vi "execute.vi"(8 "error in (no error)":errorcluster, 9 "B in":refnum<class "GenericComponent.lvclass">, 10 "A in":refnum<class "GenericComponent.lvclass">, 11 "AdapterDL111013ImagingModeToScanHead in":refnum<class "AdapterDL111013ImagingModeToScanHead.lvclass">) -> (0 "error out":errorcluster, 1 "B out":refnum<class "GenericComponent.lvclass">, 2 "A out":refnum<class "GenericComponent.lvclass">, 3 "AdapterDL111013ImagingModeToScanHead out":refnum<class "AdapterDL111013ImagingModeToScanHead.lvclass">)   [LabVIEW 2010, in "AdapterDL111013ImagingModeToScanHead.lvclass"]
uses:
  AdapterDL111013ImagingModeToScanHead.lvclass
  common/classes/GenericComponent/GenericComponent/GenericComponent.lvclass
  ImagingMode/ImagingModeDL090130Frame/ImagingModeDL090130Frame/translation_mode_enum.ctl
  ScanHead/ScanHeadDL090202/ScanHeadDL090202/ScanHeadDL090202.lvclass
  ImagingMode/ImagingModeDL090130Frame/ImagingModeDL090130Frame/settings_cluster.ctl
  ImagingMode/ImagingModeDL090130Frame/ImagingModeDL090130Frame/ImagingModeDL090130Frame.lvclass
  common/xcontrols/XIntensityCompensation/XIntensityCompensation/XIntensityCompensation.xctl
  ScanHead/ScanHeadDL090202/ScanHeadDL090202/settings_cluster.ctl
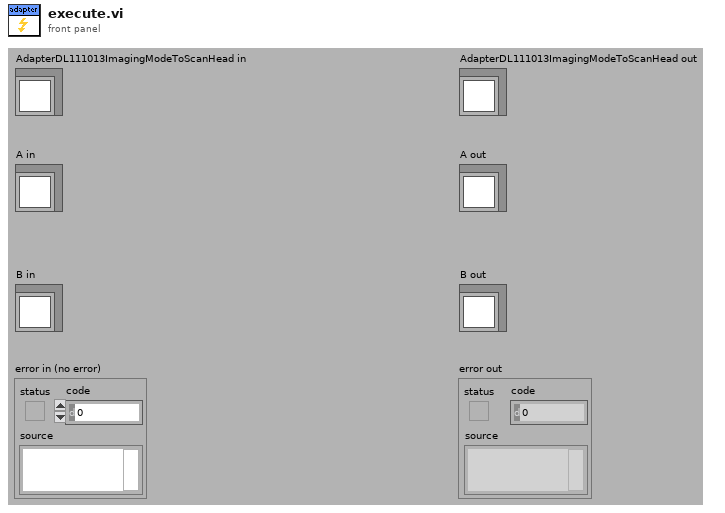
[diagram p1: front panel]
types:
  T1 = typedef "ImagingModeDL090130Frame.lvclass/translation_mode_enum.ctl" = enum16{"scanHead", "stage"}
  T2 = typedef "ImagingModeDL090130Frame.lvclass/settings_cluster.ctl" = cluster{"FrameSettings":cluster{"ResolutionX":i32, "ResolutionY":i32, "AspectRatioX":dbl, "AspectRatioY":dbl, "FrameScanRate":dbl[unit]}, "StackSettings":cluster{"Frames":i32, "AveragingRepetitions":i32, "StepSize":dbl[unit], "ReturnToOrigin":bool, "translation mode":T1, "depth/intensity points":cluster{"depth":dbl[unit], "intensity":dbl}[]}}
  T3 = typedef "ScanHeadDL090202.lvclass/settings_cluster.ctl" = cluster{"Zoom":dbl, "Intensity":dbl, "AngleZ":dbl[unit], "AngleX":dbl[unit], "OffsetX":dbl[unit], "OffsetY":dbl[unit], "OffsetZ":dbl[unit], "ScatteringLength":dbl[unit], "ScannerDelayX":i32, "ScannerDelayY":i32, "ScannerDelayZ":i32}
  T4 = typedef "ImagingModeDL090130Frame.lvclass/control_refs.ctl" = cluster{"resolution controls":cluster{"x pixels":refnum<vi>, "y pixels":refnum<vi>, "ratio x factor":refnum<vi>, "ratio y factor":refnum<vi>}, "speed controls":cluster{"pixel dwell time":refnum<vi>, "line scan time":refnum<vi>, "frame rate":refnum<vi>}, "number of frames controls":cluster{"# of frames":refnum<vi>, "duration":refnum<vi>, "# of repetitions":refnum<vi>}, "current value indicators":cluster{"frame #":refnum<vi>, "repetition #":refnum<vi>, "offset":refnum<vi>}, "step controls":cluster{"step size":refnum<vi>, "return to origin?":refnum<vi>, "translation mode":refnum<vi>, "XIntensityCompensation":refnum<vi>}, "settings":refnum<vi>, "defineButton":refnum<vi>}
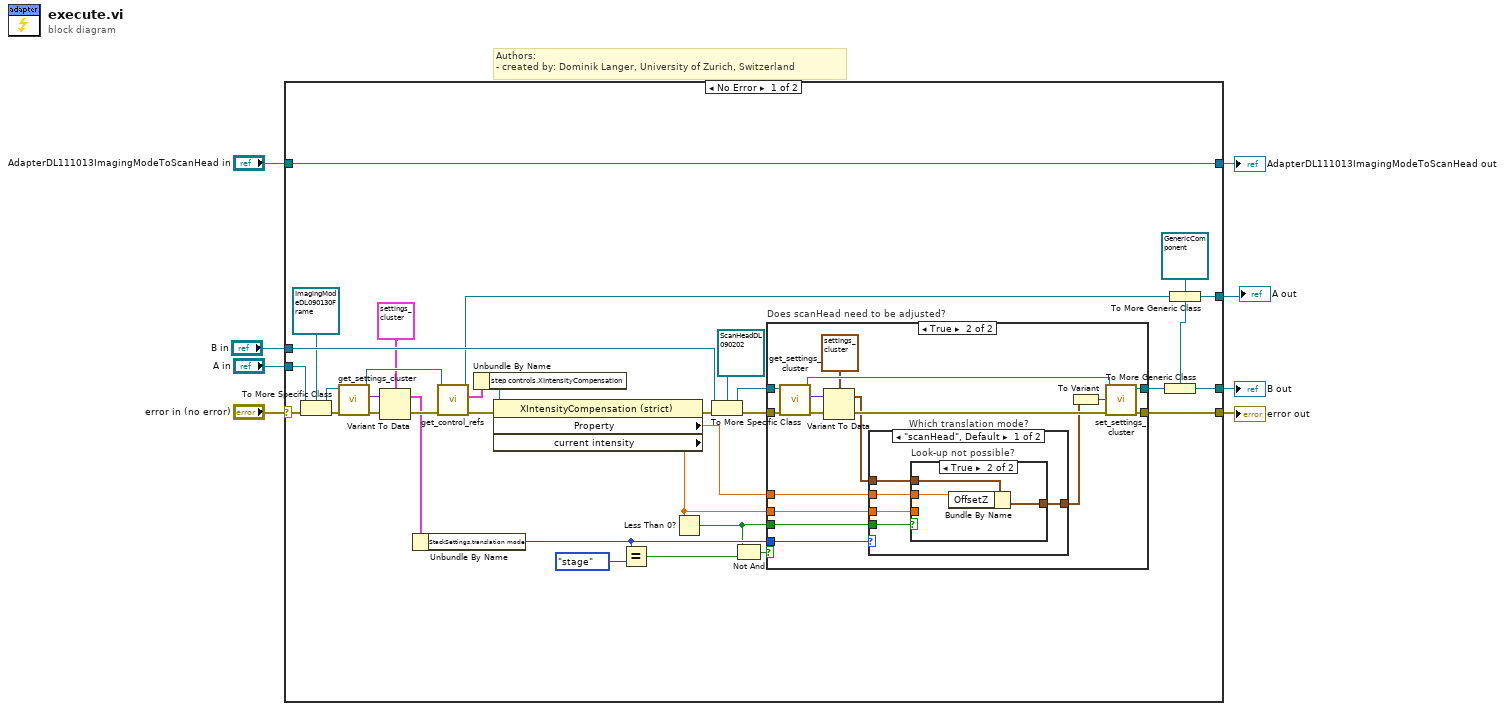
[diagram p0: block diagram]
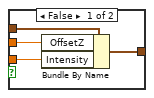
[diagram p3: hidden frame]
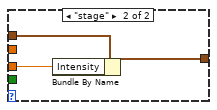
[diagram p4: hidden frame]
diagram:
  # "Authors: \n- created by: Dominik Langer, University of Zurich, Switzerland"
  n1 = case shown="No Error" "error in (no error)" {
    selector: "error in (no error)" -> [w41 w77]
    tunnel: "A in" -> [w40 w76]
    tunnel: "AdapterDL111013ImagingModeToScanHead in" -> [w39 w78]
    tunnel: [w39 w78] -> w5
    tunnel: "B in" -> [w38 w75]
    tunnel: [w27 w77] -> w3
    tunnel: [w36 w75] -> w2
    tunnel: [w35 w76] -> w1
    frame No Error {
      w37 = refnum<class "GenericComponent.lvclass"> refnum ("GenericComponent.lvclass")
      n2 = To More Specific Class(target class=refnum<class "ImagingModeDL090130Frame.lvclass"> refnum ("ImagingModeDL090130Frame.lvclass"), reference=w40, error in=w41) -> (specific class reference=w20:refnum<class "ImagingModeDL090130Frame.lvclass">, error out=w22:errorcluster)
      n3 = call-dynamic "get_settings_cluster.vi"("error in (no error)"=w22, "ImagingModeDL090130Frame in"=w20) -> ("error out"=w23:errorcluster, "settings cluster"=w19:variant, "ImagingModeDL090130Frame out"=w18:refnum<class "ImagingModeDL090130Frame.lvclass">)  [unwired: 7 in]
      n4 = Variant To Data(error in=w23, Variant=w19, type=T2 {"FrameSettings"={"ResolutionX"=0, "ResolutionY"=0, "AspectRatioX"=0.0, "AspectRatioY"=0.0, "FrameScanRate"=0.0}, "StackSettings"={"Frames"=0, "AveragingRepetitions"=0, "StepSize"=0.0, "ReturnToOrigin"=FALSE, "translation mode"=enum."scanHead", "depth/intensity points"=[]}} ("settings")) -> (error out=w21:errorcluster, data=w16:T2)
      n5 = Unbundle By Name(w16) -> ("StackSettings.translation mode"=w13:T1)
      n6 = call-dynamic "get_control_refs.vi"("error in (no error)"=w21, "ImagingModeDL090130Frame in"=w18) -> ("error out"=w32:errorcluster, "control refs"=w31:T4, "ImagingModeDL090130Frame out"=w29:refnum<class "ImagingModeDL090130Frame.lvclass">)  [unwired: 7 in]
      n7 = Unbundle By Name(w31) -> ("step controls.XIntensityCompensation"=w33:refnum<vi>)
      n8 = property class="XIntensityCompensation (strict)"(reference=w33, error in=w32) -> (error out=w30:errorcluster, "Property"=w24:dbl[unit], "current intensity"=w14:dbl)  [unwired: 1 out]
      n9 = Equal?(x=w13, y=translation_mode_enum."stage") -> (x = y?=w11:bool)
      n10 = Less Than 0?(x=w14) -> (x < 0?=w9:bool)
      n11 = To More Specific Class(target class=refnum<class "ScanHeadDL090202.lvclass"> refnum ("ScanHeadDL090202.lvclass"), reference=w38, error in=w30) -> (specific class reference=w26:refnum<class "ScanHeadDL090202.lvclass">, error out=w25:errorcluster)
      n12 = Not And(1:w11, 2:w9) -> (0:w10:bool)
      n13 = case "Does scanHead need to be adjusted?" shown="True" w10 {
        tunnel: [w42 w59] -> w28
        tunnel: [w43 w58] -> w27
        tunnel: w26 -> [w42 w57]
        tunnel: w25 -> [w43 w54]
        tunnel: w24 -> [_ w49]
        tunnel: w13 -> [_ w47]
        tunnel: w14 -> [_ w45]
        tunnel: w9 -> [_ w44]
        frame False {
        }
        frame True {
          n14 = call-dynamic "get_settings_cluster.vi"("error in (no error)"=w54, "ScanHeadDL090202 in"=w57) -> ("error out"=w55:errorcluster, "settings cluster"=w52:variant, "ScanHeadDL090202 out"=w56:refnum<class "ScanHeadDL090202.lvclass">)  [unwired: 7 in]
          n15 = Variant To Data(error in=w55, Variant=w52, type=T3 {"Zoom"=0.0, "Intensity"=0.0, "AngleZ"=0.0, "AngleX"=0.0, "OffsetX"=0.0, "OffsetY"=0.0, "OffsetZ"=0.0, "ScatteringLength"=0.0, "ScannerDelayX"=0, "ScannerDelayY"=0, "ScannerDelayZ"=0} ("settings")) -> (error out=w53:errorcluster, data=w48:T3)
          n16 = case "Which translation mode?" shown="\"scanHead\", Default" w47 {
            tunnel: [w64 w72] -> w50
            tunnel: w45 -> [w61 w73]
            tunnel: w49 -> [w63 _]
            tunnel: w48 -> [w62 w74]
            tunnel: w44 -> [w60 _]
            frame "scanHead", Default {
              n17 = case "Look-up not possible?" shown="True" w60 {
                tunnel: [w68 w71] -> w64
                tunnel: w63 -> [w67 w69]
                tunnel: w62 -> [w66 w70]
                tunnel: w61 -> [w65 _]
                frame False {
                  n18 = Bundle By Name(cluster=w66, "OffsetZ"=w67, "Intensity"=w65) -> (w68:T3)
                }
                frame True {
                  n19 = Bundle By Name(cluster=w70, "OffsetZ"=w69) -> (w71:T3)
                }
              }
            }
            frame "stage" {
              n20 = Bundle By Name(cluster=w74, "Intensity"=w73) -> (w72:T3)
            }
          }
          n21 = To Variant(anything=w50) -> (Variant=w51:variant)
          n22 = call-dynamic "set_settings_cluster.vi"("error in (no error)"=w53, "settings cluster in"=w51, "ScanHeadDL090202 in"=w56) -> ("error out"=w58:errorcluster, "ScanHeadDL090202 out"=w59:refnum<class "ScanHeadDL090202.lvclass">)  [unwired: 7 in]
        }
      }
      n23 = To More Generic Class(target class=w37, reference=w28) -> (generic class reference=w36:refnum<class "GenericComponent.lvclass">)
      n24 = To More Generic Class(target class=w37, reference=w29) -> (generic class reference=w35:refnum<class "GenericComponent.lvclass">)
    }
    frame Error {
    }
  }
  "error out" <- w3
  "AdapterDL111013ImagingModeToScanHead out" <- w5
  "A out" <- w1
  "B out" <- w2
